vi "Text To Data.vi"(0 "type descriptor":i16[](array[numeric]) format="%x", 7 "text":string, 11 "error in (no error)":errorcluster) -> (8 "flat data":string, 15 "error out":errorcluster)   [LabVIEW 2012]
uses:
  subvis/private/LuaVIEW Push (string).vi
  subvis/private/re_LuaVIEW Pull (flat data).vi
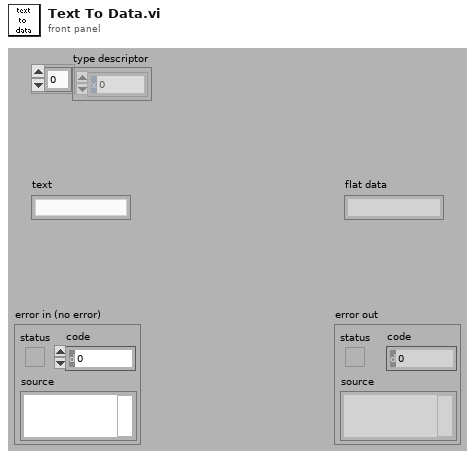
[diagram p1: front panel]
types:
  T1 = typedef "t_LuaVIEW Reference.ctl" = refnum<k1>
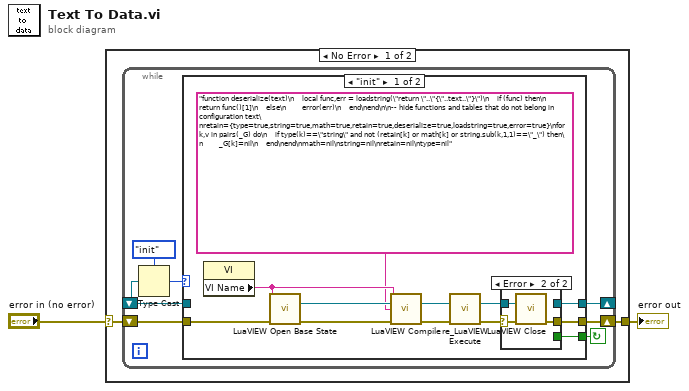
[diagram p0: block diagram]
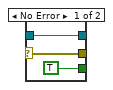
[diagram p2: hidden frame]
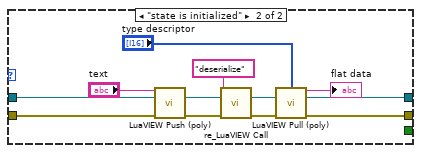
[diagram p3: hidden frame]
diagram:
  n1 = case shown="No Error" "error in (no error)" {
    selector: "error in (no error)" -> [w3 w42]
    tunnel: [w4 w42] -> w2
    frame No Error {
      n2 = while {
        shift-right: [w10] -> _
        shift-left: _ -> [w8]
        shift-right: [w9] -> w4
        shift-left: w3 -> [w11]
        stop <- w5 continue-if-true
        n3 = Type Cast(type=enum32{"init", "state is initialized"}."init", x=w8) -> (*(type *) &x=w6:enum32{"init", "state is initialized"})
        n4 = case shown="\"init\"" w6 {
          tunnel: w11 -> [w23 w41]
          tunnel: [w14 w30] -> w10
          tunnel: [w13 w39] -> w9
          tunnel: w8 -> [_ w40]
          tunnel: [w12 _] -> w5
          frame "init" {
            n5 = property class="VI"() -> ("VI Name"=w19:string)  [unwired: 2 in, 2 out]
            n6 = call "LuaVIEW Open Base State.vi"("close identifier (none)"=w19, "error in (no error)"=w23) -> ("LuaVIEW reference"=w21:T1, "error out"=w18:errorcluster)  [unwired: 12 in]
            n7 = call "LuaVIEW Compile.vi"("script name"=w19, "LuaVIEW reference in"=w21, "script"="function deserialize(text)\n    local func,err = loadstring(\"return \"..\"{\"..text..\"}\")\n    if (func) then\n        return func()[1]\n    else\n        error(err)\n    end\nend\n\n-- hide functions and tables that do not belong in configuration text\nretain={type=true,string=true,math=true,retain=true,deserialize=true,loadstring=true,error=true}\nfor k,v in pairs(_G) do\n    if type(k)==\"string\" and not (retain[k] or math[k] or string.sub(k,1,1)==\"_\") then\n        _G[k]=nil\n    end\nend\nmath=nil\nstring=nil\nretain=nil\ntype=nil", "error in (no error)"=w18) -> ("LuaVIEW reference out"=w20:T1, "error out"=w22:errorcluster)  [unwired: 10 in]
            n8 = call "re_LuaVIEW Execute.vi"("LuaVIEW reference in"=w20, "error in (no error)"=w22) -> ("LuaVIEW reference out"=w15:T1, "error out"=w16:errorcluster)  [unwired: 12 in]
            n9 = case shown="Error" w16 {
              selector: w16 -> [w25 w29]
              tunnel: w15 -> [w26 w28]
              tunnel: [w25 w27] -> w13
              tunnel: [w26 _] -> w14
              tunnel: [TRUE _] -> w12
              frame No Error {
              }
              frame Error {
                n10 = call "LuaVIEW Close.vi"("LuaVIEW reference"=w28, "error in (no error)"=w29) -> ("dup error"=w27:errorcluster)  [unwired: 13 in]
              }
            }
          }
          frame "state is initialized" {
            n11 = call-poly "LuaVIEW Push (poly).vi"("string"="text", "LuaVIEW reference in"=w40, "error in (no error)"=w41) -> ("LuaVIEW reference out"=w37:T1, "error out"=w38:errorcluster)  [unwired: 11 in]
            n12 = call "re_LuaVIEW Call.vi"("function name"="deserialize", "LuaVIEW reference in"=w37, "error in (no error)"=w38) -> ("LuaVIEW reference out"=w34:T1, "error out"=w35:errorcluster)  [unwired: 11 in]
            n13 = call-poly "LuaVIEW Pull (poly).vi"("type descriptor"="type descriptor", "LuaVIEW reference in"=w34, "error in (no error)"=w35) -> ("flat data"=→"flat data":string, "LuaVIEW reference out"=w30:T1, "error out"=w39:errorcluster)  [unwired: 10 in]
          }
        }
      }
    }
    frame Error {
    }
  }
  "error out" <- w2
